vi "Example_AOU_AWG_Array_Int16.vi"() -> ()   [LabVIEW 2013]
uses:
  <vilib>/Signadyne/Wave/base/waveformLoadInt16.vi
panel:
  out "Points":i32
  out "Points >=30":bool[](array[boolean])
  in  "AWG":u32
  in  "Run":bool
  in  "waveformType":i32(ring) items=["Analog"=0, "IQ"=2, "IQ (polar)"=3]
  out "errorOut":errorcluster
  in  "Close":bool
  in  "Prescaler":u32
  in  "Cycles":u32
  in  "Start Delay":u32
  in  "Trigger Mode":T1(ring)
  in  "nSlot":i32=7
  in  "nChassis":i32=1
  in  "partNumber":string="SD-PXE-AOU-H0002-128"
  # "Module Under Test"
  # "AWG Parameters"
  # "AWG Data"
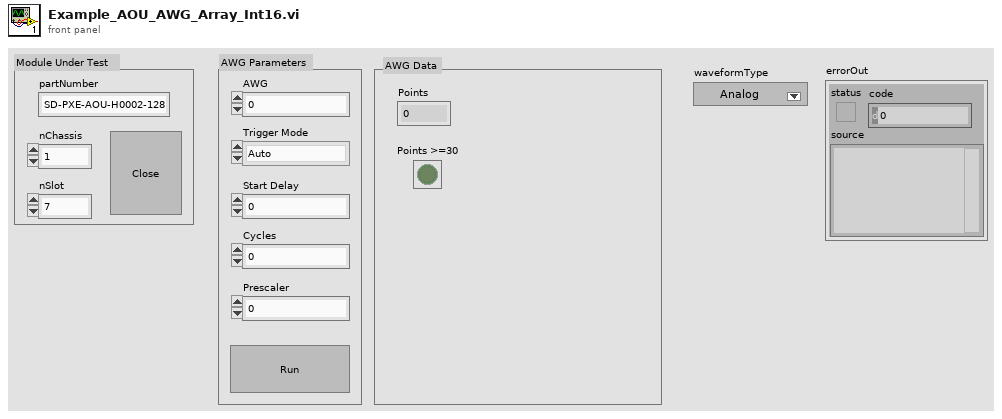
[diagram p1: front panel]
types:
  T1 = enum32{"Auto", "VI/HVI Trigger", "External Trigger"}
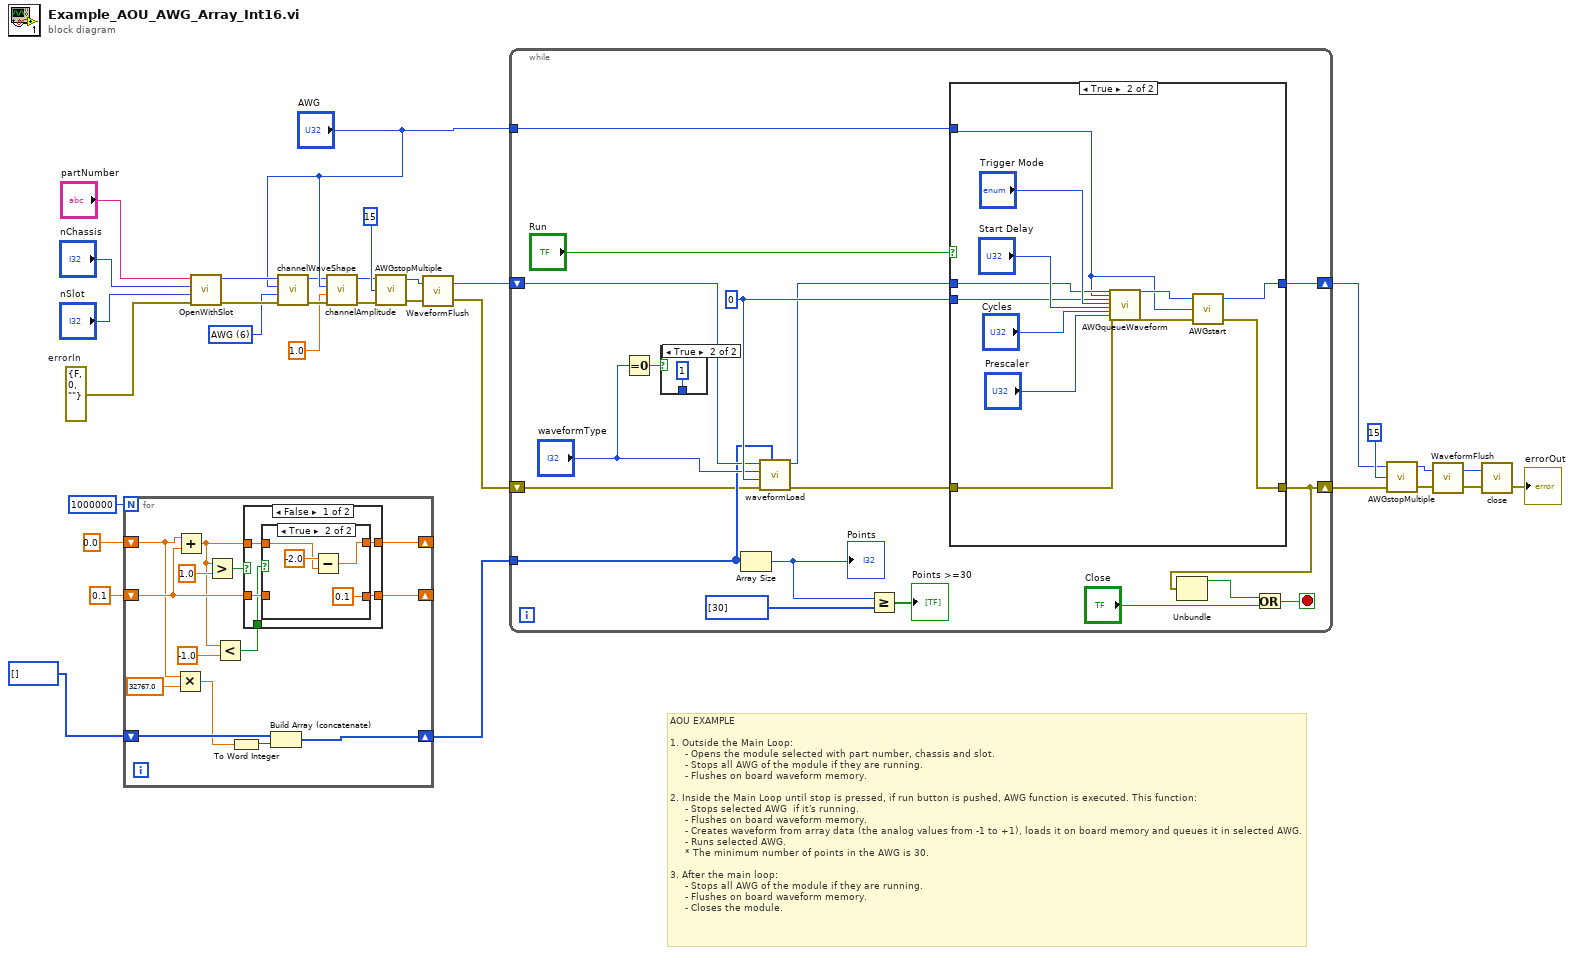
[diagram p0: block diagram]
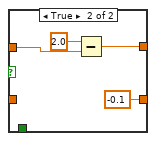
[diagram p3: hidden frame]
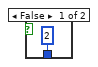
[diagram p4: hidden frame]
diagram:
  w12 = 6 items=["None"=-1, "Sinusoidal"=1, "Triangular"=2, "Sawtooth"=3, "Square"=4, "DC"=5, "AWG"=6] ("waveShape")
  w16 = errorcluster {"status"=FALSE, "code"=0, "source"=""}  # errorIn
  # "AOU EXAMPLE\n\n1. Outside the Main Loop:\n     - Opens the module selected with part number, chassis and slot.\n     - Stops all AWG of the module if they are running.\n     - Flushes on board waveform memory.\n\n2. Inside the Main Loop until stop is pressed, if run button is pushed, AWG function is executed. This function:\n     - Stops selected AWG  if it's running.\n     - Flushes on board waveform memory.\n     - Creates waveform from array data (the analog values from -1 to +1), loads it on board memory and queues it in selected AWG.\n     - Runs selected AWG.\n     * The minimum number of points in the AWG is 30.  \n\n3. After the main loop:\n     - Stops all AWG of the module if they are running.\n     - Flushes on board waveform memory.\n     - Closes the module."
  n1 = for {
    N: 1000000 -> [_]
    shift-right: [w43] -> _
    shift-left: 0.0 -> [w37]
    shift-right: [w42] -> _
    shift-left: 0.1 -> [w41]
    shift-right: [w34] -> w1
    shift-left: i16[] [] ("waveformData") -> [w35]
    n2 = Multiply(x=w37, y=32767.0) -> (x*y=w32:dbl)
    n3 = Add(x=w37, y=w41) -> (x+y=w38:dbl)
    n4 = Greater?(x=w38, y=1.0) -> (0:w45:bool)
    n5 = Less?(x=w38, y=-1.0) -> (x < y?=w40:bool)
    n6 = To Word Integer(number=w32) -> (16bit integer=w33:i16)
    n7 = case shown="False" w45 {
      tunnel: w38 -> [w50 w60]
      tunnel: [w47 w58] -> w43
      tunnel: w41 -> [w49 _]
      tunnel: [w48 -0.1] -> w42
      tunnel: w40 -> [w46 _]
      frame False {
        n8 = case shown="True" w46 {
          tunnel: w50 -> [w51 w53]
          tunnel: [w52 0.1] -> w48
          tunnel: w49 -> [w52 _]
          tunnel: [w51 w54] -> w47
          frame False {
          }
          frame True {
            n9 = Subtract(x=-2.0, y=w53) -> (x-y=w54:dbl)
          }
        }
      }
      frame True {
        n10 = Subtract(x=2.0, y=w60) -> (x-y=w58:dbl)
      }
    }
    n11 = Build Array (concatenate)(w35, w33) -> (w34:i16[])
  }
  n12 = call <vilib>:"OpenWithSlot.vi"("errorIn"=w16, "nSlot"="nSlot", "nChassis"="nChassis", "partNumber"="partNumber") -> ("errorOut"=w13:errorcluster, "moduleID"=w14:i32)  [unwired: 2 in]
  n13 = call <vilib>:"channelWaveShape.vi"("errorIn"=w13, "waveShape"=w12, "nChannel"="AWG", "moduleID"=w14) -> ("errorOut"=w11:errorcluster, "moduleIDOut"=w8:i32)  [unwired: 2 in]
  n14 = call <vilib>:"channelAmplitude.vi"("errorIn"=w11, "amplitude"=1.0, "nChannel"="AWG", "moduleID"=w8) -> ("errorOut"=w10:errorcluster, "moduleIDOut"=w7:i32)  [unwired: 2 in]
  n15 = call <vilib>:"AWGstopMultiple.vi"("errorIn"=w10, "AWGmask"=15, "moduleID"=w7) -> ("errorOut"=w19:errorcluster, "moduleIDOut"=w18:i32)  [unwired: 1 in]
  n16 = call <vilib>:"WaveformFlush.vi"("errorIn"=w19, "moduleID"=w18) -> ("errorOut"=w28:errorcluster, "moduleIDOut"=w29:i32)
  n17 = while {
    shift-right: [w73] -> w23
    shift-left: w28 -> [w61]
    shift-right: [w77] -> w15
    shift-left: w29 -> [w66]
    tunnel: "AWG" -> [w71]
    tunnel: w1 -> [w62]
    stop <- w76 stop-if-true
    w67 = 0 ("waveformNumber")
    n18 = Equal To 0?(x="waveformType") -> (x = 0?=w72:bool)
    n19 = case shown="True" w72 {
      tunnel: [2 1] -> _
      frame False {
      }
      frame True {
      }
    }
    n20 = Array Size(array=w62) -> (size(s)=w68:i32)
    "Points" <- w68
    n21 = call-poly <vilib>:"waveformLoad.vi"("waveformData"=w62, "errorIn"=w61, "waveformNumber"=w67, "waveformType"="waveformType", "moduleID"=w66) -> ("errorOut"=w63:errorcluster, "moduleIDOut"=w64:i32)  [unwired: 2 in, 1 out]
    n22 = Greater Or Equal?(x=w68, y=i32[] [30]) -> (x >= y?=→"Points >=30":bool[])
    n23 = case shown="True" "Run" {
      tunnel: w64 -> [w82 w84]
      tunnel: w63 -> [w81 w90]
      tunnel: [w81 w85] -> w73
      tunnel: [w82 w87] -> w77
      tunnel: w71 -> [_ w83]
      tunnel: w67 -> [_ w89]
      frame False {
      }
      frame True {
        n24 = call <vilib>:"AWGqueueWaveform.vi"("moduleID"=w84, "nAWG"=w83, "waveformNumber"=w89, "triggerMode"="Trigger Mode", "startDelay"="Start Delay", "cycles"="Cycles", "prescaler"="Prescaler", "errorIn"=w90) -> ("moduleIDOut"=w88:i32, "errorOut"=w86:errorcluster)  [unwired: 18 in]
        n25 = call <vilib>:"AWGstart.vi"("errorIn"=w86, "nAWG"=w83, "moduleID"=w88) -> ("errorOut"=w85:errorcluster, "moduleIDOut"=w87:i32)  [unwired: 1 in]
      }
    }
    n26 = Unbundle(w73) -> ("status"=w75:bool)  [unwired: 2 out]
    n27 = Or(x=w75, y="Close") -> (x .or. y?=w76:bool)
  }
  n28 = call <vilib>:"AWGstopMultiple.vi"("errorIn"=w23, "AWGmask"=15, "moduleID"=w15) -> ("errorOut"=w22:errorcluster, "moduleIDOut"=w21:i32)  [unwired: 1 in]
  n29 = call <vilib>:"WaveformFlush.vi"("errorIn"=w22, "moduleID"=w21) -> ("errorOut"=w26:errorcluster, "moduleIDOut"=w25:i32)
  n30 = call <vilib>:"close.vi"("errorIn"=w26, "moduleID"=w25) -> ("errorOut"=→"errorOut":errorcluster)  [unwired: 1 in]
